vi "desaccade_v2.vi"(10 "Sample Rate":dbl=500.0 format="%.2f", 11 "Velocity Data IN":dbl[][](array[numeric])) -> ()   [LabVIEW 2016]
uses:
  <vilib>/Analysis/3filter.llb/Savitzky-Golay Filter (DBL).vi
  comm.lvlib
  <vilib>/Analysis/NI_AALPro.lvlib
  <vilib>/Analysis/NI_AALBase.lvlib
  <vilib>/Analysis/NI_AAL_SigProc.lvlib
panel:
  out "Waveform Graph 3":dbl[][](graph)
  out "Waveform Graph 2":dbl[](graph)
  out "Waveform Graph":dbl[][](graph)
  in  "Impulse Positions":T1(array[cluster])=[{"Start"=-31, "End"=518, "Impulse Plane"=enum."Other", "Impulse Direction +ve?"=TRUE, "Time offset"=0, "Amplitude offset"=0.0}, {"Start"=369, "End"=913, "Impulse Plane"=enum."Other", "Impulse Direction +ve?"=TRUE, "Time offset"=0, "Amplitude offset"=0.0}, {"Start"=570, "End"=1018, "Impulse Plane"=enum."Other", "Impulse Direction +ve?"=FALSE, "Time offset"=0, "Amplitude offset"=0.0}, {"Start"=770, "End"=1311, "Impulse Plane"=enum."Other", "Impulse Direction +ve?"=TRUE, "Time offset"=0, "Amplitude offset"=0.0}, {"Start"=969, "End"=1417, "Impulse Plane"=enum."Other", "Impulse Direction +ve?"=FALSE, "Time offset"=0, "Amplitude offset"=0.0}, {"Start"=1170, "End"=1708, "Impulse Plane"=enum."Other", "Impulse Direction +ve?"=TRUE, "Time offset"=0, "Amplitude offset"=0.0}, {"Start"=1371, "End"=1819, "Impulse Plane"=enum."Other", "Impulse Direction +ve?"=FALSE, "Time offset"=0, "Amplitude offset"=0.0}, {"Start"=1570, "End"=2104, "Impulse Plane"=enum."Other", "Impulse Direction +ve?"=TRUE, "Time offset"=0, "Amplitude offset"=0.0}, {"Start"=1770, "End"=2218, "Impulse Plane"=enum."Other", "Impulse Direction +ve?"=FALSE, "Time offset"=0, "Amplitude offset"=0.0}, {"Start"=1971, "End"=2508, "Impulse Plane"=enum."Other", "Impulse Direction +ve?"=TRUE, "Time offset"=0, "Amplitude offset"=0.0}, {"Start"=2171, "End"=2619, "Impulse Plane"=enum."Other", "Impulse Direction +ve?"=FALSE, "Time offset"=0, "Amplitude offset"=0.0}, {"Start"=2370, "End"=2917, "Impulse Plane"=enum."Other", "Impulse Direction +ve?"=TRUE, "Time offset"=0, "Amplitude offset"=0.0}, {"Start"=2571, "End"=3019, "Impulse Plane"=enum."Other", "Impulse Direction +ve?"=FALSE, "Time offset"=0, "Amplitude offset"=0.0}, {"Start"=2771, "End"=3308, "Impulse Plane"=enum."Other", "Impulse Direction +ve?"=TRUE, "Time offset"=0, "Amplitude offset"=0.0}, {"Start"=2970, "End"=3418, "Impulse Plane"=enum."Other", "Impulse Direction +ve?"=FALSE, "Time offset"=0, "Amplitude offset"=0.0}, {"Start"=3172, "End"=3715, "Impulse Plane"=enum."Other", "Impulse Direction +ve?"=TRUE, "Time offset"=0, "Amplitude offset"=0.0}, {"Start"=3372, "End"=3820, "Impulse Plane"=enum."Other", "Impulse Direction +ve?"=FALSE, "Time offset"=0, "Amplitude offset"=0.0}, {"Start"=3572, "End"=4107, "Impulse Plane"=enum."Other", "Impulse Direction +ve?"=TRUE, "Time offset"=0, "Amplitude offset"=0.0}, {"Start"=3772, "End"=4220, "Impulse Plane"=enum."Other", "Impulse Direction +ve?"=FALSE, "Time offset"=0, "Amplitude offset"=0.0}, {"Start"=3972, "End"=4512, "Impulse Plane"=enum."Other", "Impulse Direction +ve?"=TRUE, "Time offset"=0, "Amplitude offset"=0.0}, {"Start"=4172, "End"=4620, "Impulse Plane"=enum."Other", "Impulse Direction +ve?"=FALSE, "Time offset"=0, "Amplitude offset"=0.0}, {"Start"=4373, "End"=4920, "Impulse Plane"=enum."Other", "Impulse Direction +ve?"=TRUE, "Time offset"=0, "Amplitude offset"=0.0}, {"Start"=4572, "End"=5020, "Impulse Plane"=enum."Other", "Impulse Direction +ve?"=FALSE, "Time offset"=0, "Amplitude offset"=0.0}, {"Start"=4773, "End"=5315, "Impulse Plane"=enum."Other", "Impulse Direction +ve?"=TRUE, "Time offset"=0, "Amplitude offset"=0.0}, {"Start"=4973, "End"=5421, "Impulse Plane"=enum."Other", "Impulse Direction +ve?"=FALSE, "Time offset"=0, "Amplitude offset"=0.0}, {"Start"=5173, "End"=5716, "Impulse Plane"=enum."Other", "Impulse Direction +ve?"=TRUE, "Time offset"=0, "Amplitude offset"=0.0}, {"Start"=5373, "End"=5821, "Impulse Plane"=enum."Other", "Impulse Direction +ve?"=FALSE, "Time offset"=0, "Amplitude offset"=0.0}, {"Start"=5573, "End"=6110, "Impulse Plane"=enum."Other", "Impulse Direction +ve?"=TRUE, "Time offset"=0, "Amplitude offset"=0.0}, {"Start"=5773, "End"=6221, "Impulse Plane"=enum."Other", "Impulse Direction +ve?"=FALSE, "Time offset"=0, "Amplitude offset"=0.0}, {"Start"=5972, "End"=6515, "Impulse Plane"=enum."Other", "Impulse Direction +ve?"=TRUE, "Time offset"=0, "Amplitude offset"=0.0}, {"Start"=6174, "End"=6622, "Impulse Plane"=enum."Other", "Impulse Direction +ve?"=FALSE, "Time offset"=0, "Amplitude offset"=0.0}, {"Start"=6373, "End"=6913, "Impulse Plane"=enum."Other", "Impulse Direction +ve?"=TRUE, "Time offset"=0, "Amplitude offset"=0.0}, {"Start"=6574, "End"=7022, "Impulse Plane"=enum."Other", "Impulse Direction +ve?"=FALSE, "Time offset"=0, "Amplitude offset"=0.0}, {"Start"=6774, "End"=7314, "Impulse Plane"=enum."Other", "Impulse Direction +ve?"=TRUE, "Time offset"=0, "Amplitude offset"=0.0}, {"Start"=6974, "End"=7422, "Impulse Plane"=enum."Other", "Impulse Direction +ve?"=FALSE, "Time offset"=0, "Amplitude offset"=0.0}, {"Start"=7175, "End"=7712, "Impulse Plane"=enum."Other", "Impulse Direction +ve?"=TRUE, "Time offset"=0, "Amplitude offset"=0.0}, {"Start"=7374, "End"=7822, "Impulse Plane"=enum."Other", "Impulse Direction +ve?"=FALSE, "Time offset"=0, "Amplitude offset"=0.0}, {"Start"=7574, "End"=8111, "Impulse Plane"=enum."Other", "Impulse Direction +ve?"=TRUE, "Time offset"=0, "Amplitude offset"=0.0}, {"Start"=7774, "End"=8222, "Impulse Plane"=enum."Other", "Impulse Direction +ve?"=FALSE, "Time offset"=0, "Amplitude offset"=0.0}, {"Start"=7974, "End"=8518, "Impulse Plane"=enum."Other", "Impulse Direction +ve?"=TRUE, "Time offset"=0, "Amplitude offset"=0.0}, {"Start"=8175, "End"=8623, "Impulse Plane"=enum."Other", "Impulse Direction +ve?"=FALSE, "Time offset"=0, "Amplitude offset"=0.0}, {"Start"=8375, "End"=8920, "Impulse Plane"=enum."Other", "Impulse Direction +ve?"=TRUE, "Time offset"=0, "Amplitude offset"=0.0}, {"Start"=8575, "End"=9023, "Impulse Plane"=enum."Other", "Impulse Direction +ve?"=FALSE, "Time offset"=0, "Amplitude offset"=0.0}, {"Start"=8776, "End"=9315, "Impulse Plane"=enum."Other", "Impulse Direction +ve?"=TRUE, "Time offset"=0, "Amplitude offset"=0.0}, {"Start"=8975, "End"=9423, "Impulse Plane"=enum."Other", "Impulse Direction +ve?"=FALSE, "Time offset"=0, "Amplitude offset"=0.0}, {"Start"=9176, "End"=9715, "Impulse Plane"=enum."Other", "Impulse Direction +ve?"=TRUE, "Time offset"=0, "Amplitude offset"=0.0}, {"Start"=9375, "End"=9823, "Impulse Plane"=enum."Other", "Impulse Direction +ve?"=FALSE, "Time offset"=0, "Amplitude offset"=0.0}, {"Start"=9575, "End"=10110, "Impulse Plane"=enum."Other", "Impulse Direction +ve?"=TRUE, "Time offset"=0, "Amplitude offset"=0.0}]
  in  "Desaccading Parameter":T2={"Threshold 1 [Acc]"=0.0, "Threshold 2 [% of TH1]"=0, "tolerance"=2.0, "Search WD "=0.05757575757575758, " always use TH2"=TRUE, "SD for Outliers"=3.0303030303030303, "Max time [ms]"=50.0, "Min time [ms]"=1.0, "Velocity Threshold"=0.05757575757575758} {"Velocity Threshold" scale=50.0..400.0; "SD for Outliers" scale=0.0..5.0; "Search WD" scale=0.0..0.3; "tolerance" scale=0.0..100.0; "Threshold 2 [% of TH1]" scale=0.0..100.0; "Threshold 1 [Acc]" scale=1.0..40000.0}
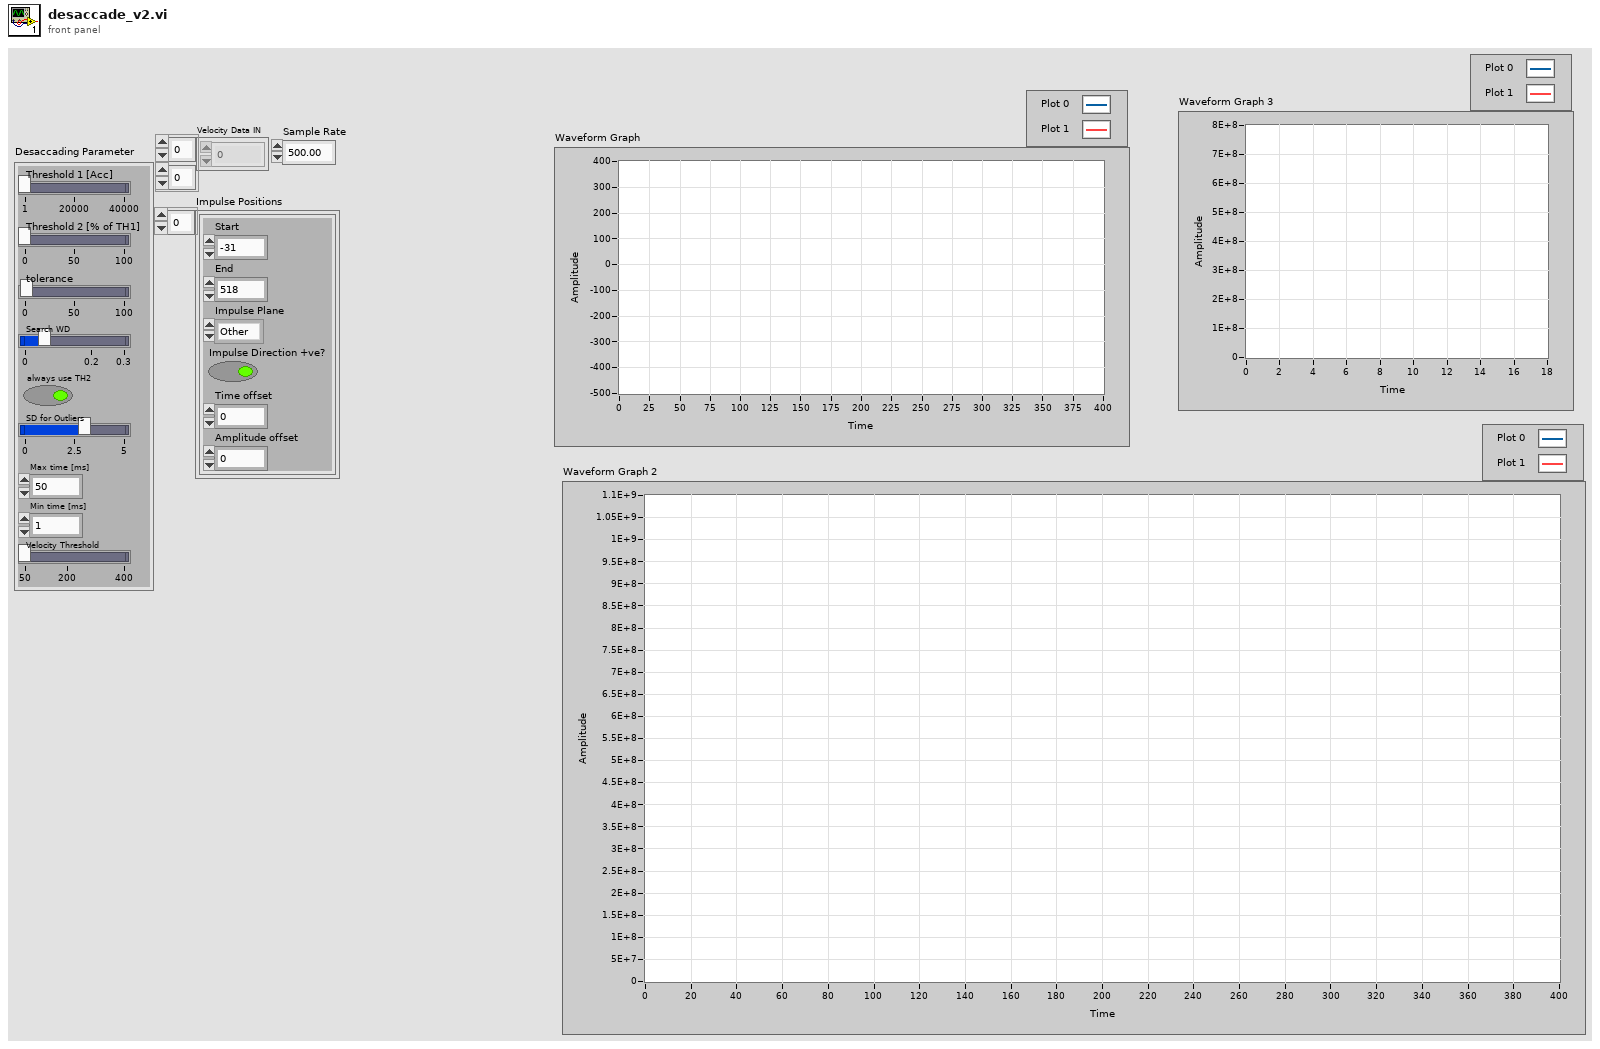
[diagram p1: front panel]
types:
  T1 = cluster{"Start":i32, "End":i32, "Impulse Plane":enum16{"Other", "Yaw", "Pitch", "Roll", "LARP", "RALP"}, "Impulse Direction +ve?":bool, "Time offset":i32, "Amplitude offset":dbl}[]
  T2 = cluster{"Threshold 1 [Acc]":dbl, "Threshold 2 [% of TH1]":i32, "tolerance":dbl, "Search WD ":dbl, " always use TH2":bool, "SD for Outliers":dbl, "Max time [ms]":dbl, "Min time [ms]":dbl, "Velocity Threshold":dbl}
  T3 = cluster{"Raw Acceleration":dbl[], "Smooth Acceleration":dbl[], "Raw Velocity":dbl[], "Smooth Velocity":dbl[]}
  T4 = cluster{"Desaccading Parameter ":cluster{"Threshold 1 [Acc]":dbl, "Threshold 2 [% of TH1]":i32, "tolerance":dbl, "Search WD ":dbl, " always use TH2":bool, "SD for Outliers":dbl, "Max time [ms]":dbl, "Min time [ms]":dbl, "Velocity Threshold":dbl}, "Impulse Positions":cluster{"Start":i32, "End":i32, "Impulse Plane":enum16{"Other", "Yaw", "Pitch", "Roll", "LARP", "RALP"}, "Impulse Direction +ve?":bool, "Time offset":i32, "Amplitude offset":dbl}[], "Velocity Data IN":dbl[][], "Impulse ID":i32, "Sample Rate":dbl, "1D Data":cluster{"Raw Acceleration":dbl[], "Smooth Acceleration":dbl[], "Raw Velocity":dbl[], "Smooth Velocity":dbl[]}, "Datapoint ID":i32, "Saccade Start-End":dbl[]}
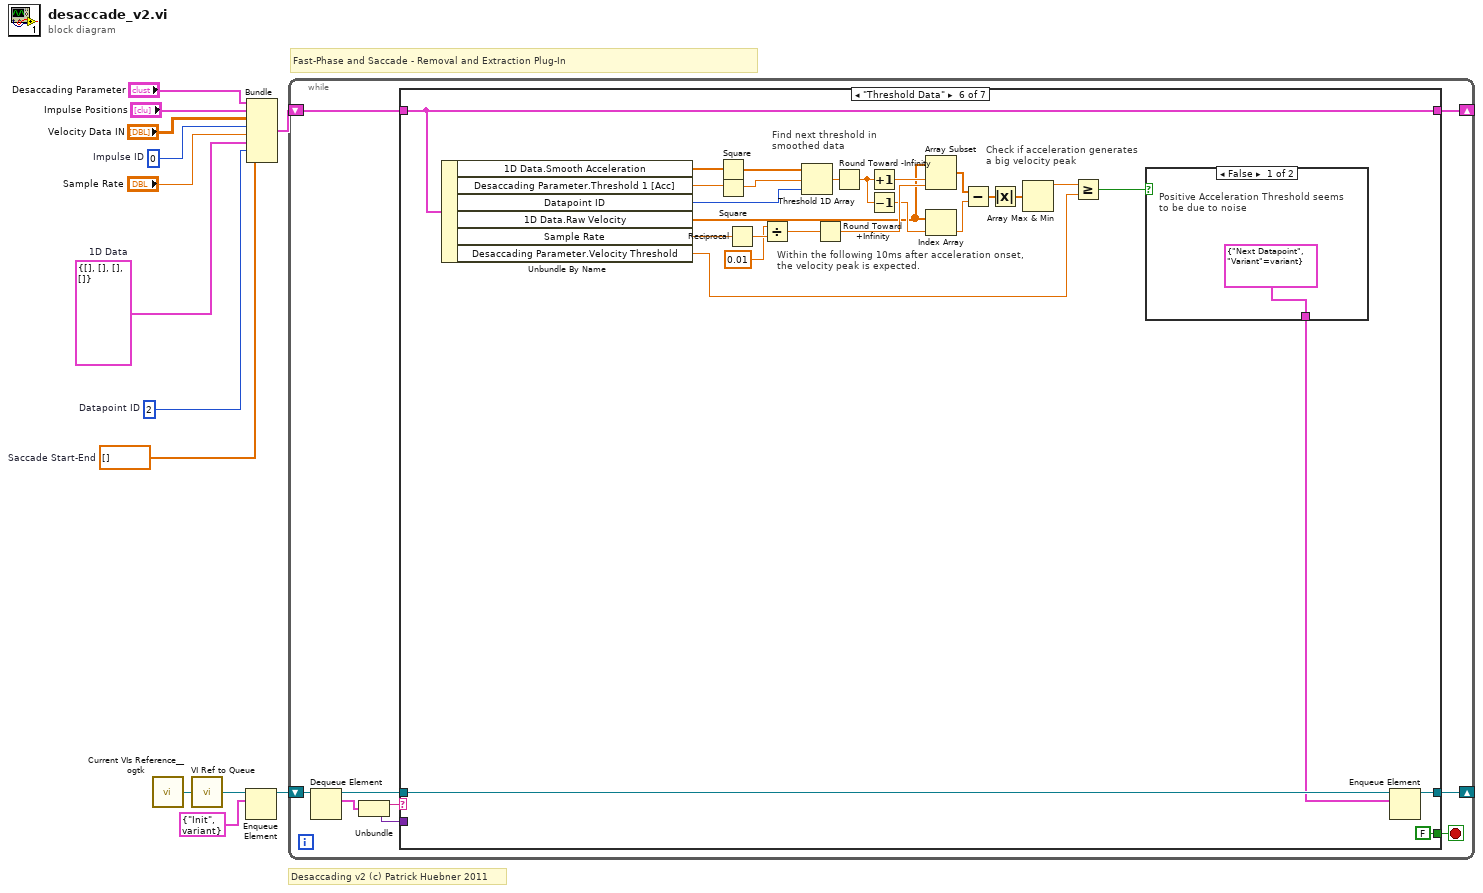
[diagram p0: block diagram]
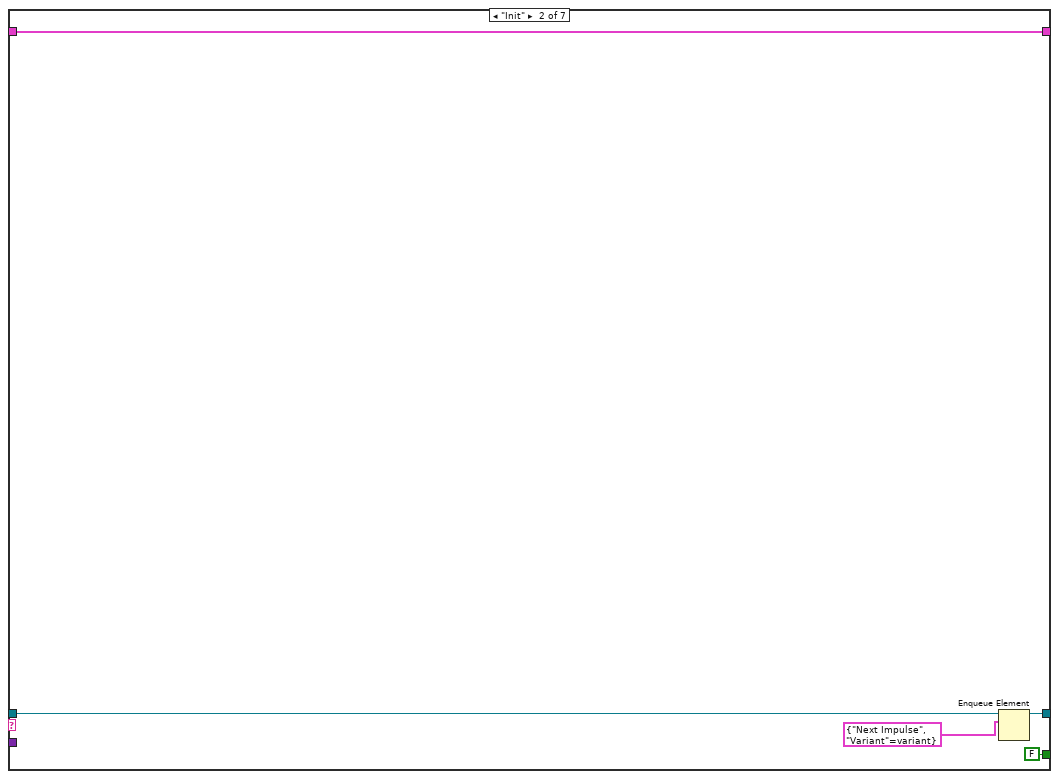
[diagram p3: hidden frame]
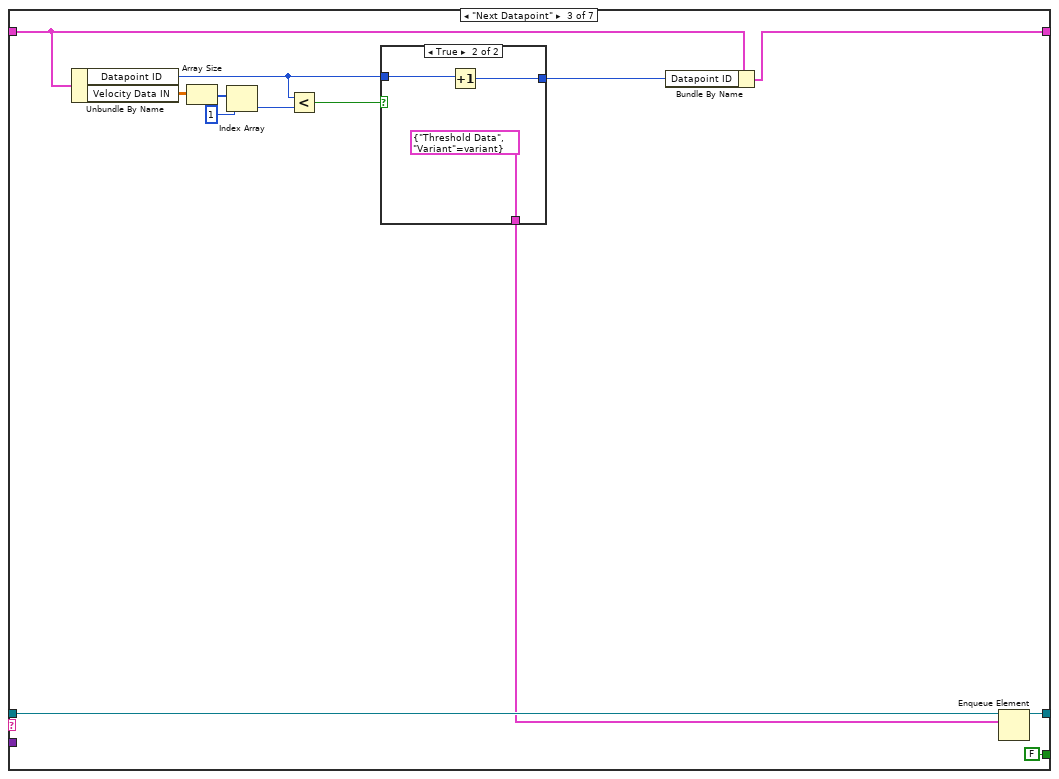
[diagram p4: hidden frame]
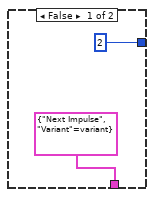
[diagram p5: hidden frame]
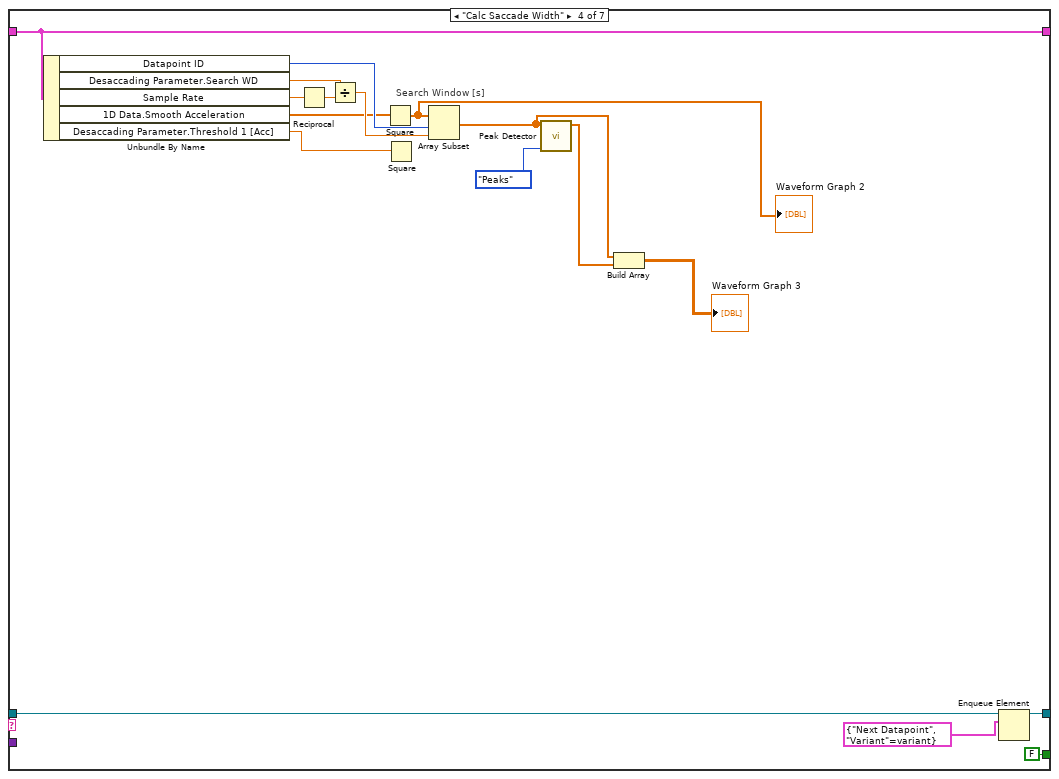
[diagram p6: hidden frame]
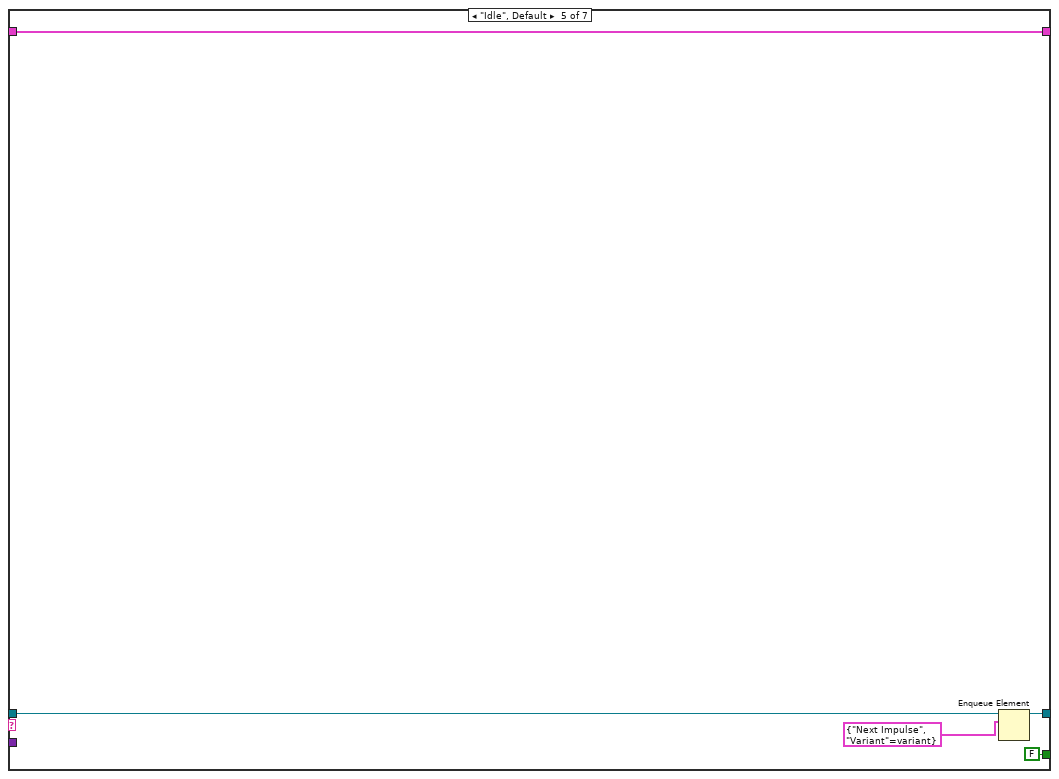
[diagram p7: hidden frame]
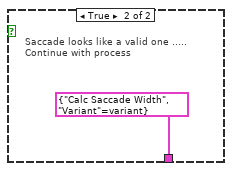
[diagram p8: hidden frame]
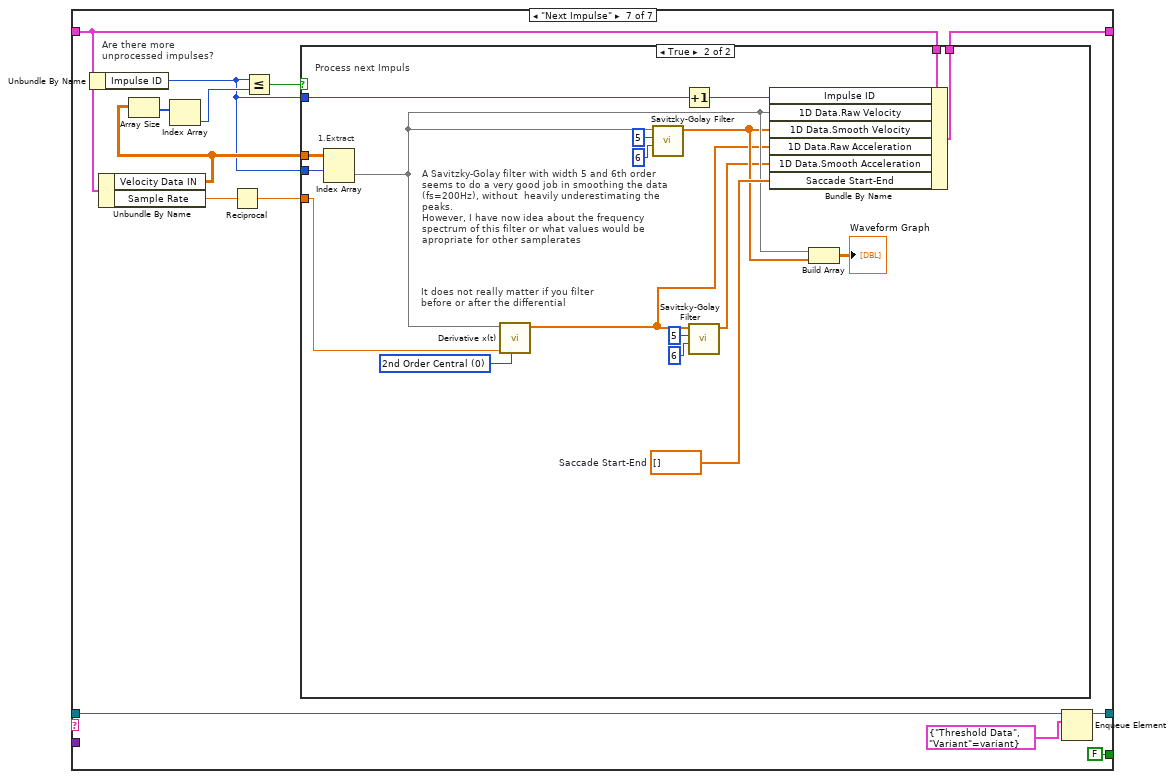
[diagram p9: hidden frame]
diagram:
  w1 = dbl[] []  # Saccade Start-End
  w2 = 2  # Datapoint ID
  w3 = T3 {"Raw Acceleration"=[], "Smooth Acceleration"=[], "Raw Velocity"=[], "Smooth Velocity"=[]}  # 1D Data
  w6 = 0  # Impulse ID
  # "Fast-Phase and Saccade - Removal and Extraction Plug-In"
  # "Desaccading v2 (c) Patrick Huebner 2011"
  n1 = call <userlib>:"Current VIs Reference__ogtk.vi"() -> ("Current VI's reference"=w13:refnum<vi>)  [unwired: 5 in]
  n2 = call "VI Ref to Queue.vi"("VI Refnum"=w13) -> ("queue out"=w12:refnum<queue>)  [unwired: 4 in]
  n3 = Enqueue Element(queue=w12, element=cluster{string, "Variant":variant} {"Init", "Variant"=variant}) -> (queue out=w10:refnum<queue>)  [unwired: 2 in, 2 out]
  n4 = Bundle("Desaccading Parameter"="Desaccading Parameter", "Impulse Positions"="Impulse Positions", "Velocity Data IN"="Velocity Data IN", "Impulse ID"=w6, "Sample Rate"="Sample Rate", "1D Data"=w3, "Datapoint ID"=w2, "Saccade Start-End"=w1) -> (w8:T4)  [unwired: 1 in]
  n5 = while {
    shift-right: [w21] -> _
    shift-left: w10 -> [w22]
    shift-right: [w15] -> _
    shift-left: w8 -> [w14]
    stop <- w16 stop-if-true
    n6 = Dequeue Element(queue=w22) -> (queue out=w20:refnum<queue>, element=w19:cluster{string, "Variant":variant})  [unwired: 2 in, 2 out]
    n7 = Unbundle(w19) -> (w18:string, "Variant"=w17:variant)
    n8 = case shown="\"Threshold Data\"" w18 {
      tunnel: [w24 w29 w42 w64 w69 w96 w111] -> w21
      tunnel: w20 -> [w24 w28 w41 w63 w68 w95 w110]
      tunnel: w17 -> [_ _ _ _ _ _ _]
      tunnel: [_ FALSE FALSE FALSE FALSE FALSE FALSE] -> w16
      tunnel: [w23 w25 w38 w60 w65 w93 w100] -> w15
      tunnel: w14 -> [w23 w25 w39 w60 w65 w93 w101]
      frame "Differentiate" {
      }
      frame "Init" {
        n9 = Enqueue Element(queue=w28, element=cluster{string, "Variant":variant} {"Next Impulse", "Variant"=variant}) -> (queue out=w29:refnum<queue>)  [unwired: 2 in, 2 out]
      }
      frame "Next Datapoint" {
        n10 = Unbundle By Name(w39) -> ("Datapoint ID"=w34:i32, "Velocity Data IN"=w36:dbl[][])
        n11 = Array Size(array=w36) -> (size(s)=w35:i32[])
        n12 = Index Array(array=w35, index=1) -> (element=w33:i32)
        n13 = Less?(x=w34, y=w33) -> (x < y?=w32:bool)
        n14 = case shown="True" w32 {
          tunnel: w34 -> [_ w47]
          tunnel: [2 w46] -> w37
          tunnel: [cluster{string, "Variant":variant} {"Next Impulse", "Variant"=variant} ("element") cluster{string, "Variant":variant} {"Threshold Data", "Variant"=variant} ("element")] -> w31
          frame False {
          }
          frame True {
            n15 = Increment(x=w47) -> (x+1=w46:i32)
          }
        }
        n16 = Bundle By Name(cluster=w39, "Datapoint ID"=w37) -> (w38:T4)
        n17 = Enqueue Element(queue=w41, element=w31) -> (queue out=w42:refnum<queue>)  [unwired: 2 in, 2 out]
      }
      frame "Calc Saccade Width" {
        # "Search Window [s]"
        n18 = Unbundle By Name(w60) -> ("Datapoint ID"=w56:i32, "Desaccading Parameter.Search WD"=w57:dbl, "Sample Rate"=w59:dbl, "1D Data.Smooth Acceleration"=w54:dbl[], "Desaccading Parameter.Threshold 1 [Acc]"=w53:dbl)
        n19 = Reciprocal(x=w59) -> (1/x=w58:dbl)
        n20 = Divide(x=w57, y=w58) -> (x/y=w55:dbl)
        n21 = Square(x=w54) -> (x^2=w51:dbl[])
        "Waveform Graph 2" <- w51
        n22 = Square(x=w53) -> ()  [unwired: 1 out]
        n23 = Array Subset(array=w51, index=w56, length=w55) -> (w49:dbl[])
        n24 = call <vilib>:"Peak Detector.vi"("peaks/valleys"=enum32{"Peaks", "Valleys"}."Peaks", "X"=w49) -> ("Locations"=w48:dbl[])  [unwired: 5 in, 4 out]
        n25 = Build Array(w49, w48) -> (→"Waveform Graph 3":dbl[][])
        n26 = Enqueue Element(queue=w63, element=cluster{string, "Variant":variant} {"Next Datapoint", "Variant"=variant}) -> (queue out=w64:refnum<queue>)  [unwired: 2 in, 2 out]
      }
      frame "Idle", Default {
        n27 = Enqueue Element(queue=w68, element=cluster{string, "Variant":variant} {"Next Impulse", "Variant"=variant}) -> (queue out=w69:refnum<queue>)  [unwired: 2 in, 2 out]
      }
      frame "Threshold Data" {
        # "Check if acceleration generates \na big velocity peak"
        # "Within the following 10ms after acceleration onset, \nthe velocity peak is expected."
        # "Find next threshold in \nsmoothed data"
        n28 = Unbundle By Name(w93) -> ("1D Data.Smooth Acceleration"=w92:dbl[], "Desaccading Parameter.Threshold 1 [Acc]"=w71:dbl, "Datapoint ID"=w89:i32, "1D Data.Raw Velocity"=w80:dbl[], "Sample Rate"=w87:dbl, "Desaccading Parameter.Velocity Threshold"=w74:dbl)
        n29 = Square(x=w92) -> (x^2=w90:dbl[])
        n30 = Square(x=w71) -> (x^2=w70:dbl)
        n31 = Reciprocal(x=w87) -> (1/x=w86:dbl)
        n32 = Divide(x=0.01 ("y"), y=w86) -> (x/y=w84:dbl)
        n33 = Threshold 1D Array(1:w89, 2:w70, 3:w90) -> (0:w91:dbl)
        n34 = Round Toward +Infinity(x=w84) -> (ceil(x): smallest int >= x=w83:dbl)
        n35 = Round Toward -Infinity(1:w91) -> (0:w82:dbl)
        n36 = Increment(x=w82) -> (x+1=w88:dbl)
        n37 = Decrement(x=w82) -> (x-1=w81:dbl)
        n38 = Array Subset(array=w80, index=w88, length=w83) -> (w79:dbl[])
        n39 = Index Array(array=w80, index=w81) -> (element=w78:dbl)
        n40 = Subtract(x=w79, y=w78) -> (x-y=w77:dbl[])
        n41 = Absolute Value(x=w77) -> (abs(x)=w76:dbl[])
        n42 = Array Max & Min(array=w76) -> (max value=w75:dbl)  [unwired: 3 out]
        n43 = Greater Or Equal?(x=w75, y=w74) -> (x >= y?=w73:bool)
        n44 = case shown="False" w73 {
          tunnel: [cluster{string, "Variant":variant} {"Next Datapoint", "Variant"=variant} ("element") cluster{string, "Variant":variant} {"Calc Saccade Width", "Variant"=variant} ("element")] -> w72
          frame False {
            # "Positive Acceleration Threshold seems\nto be due to noise"
          }
          frame True {
            # "Saccade looks like a valid one .....\nContinue with process"
          }
        }
        n45 = Enqueue Element(queue=w95, element=w72) -> (queue out=w96:refnum<queue>)  [unwired: 2 in, 2 out]
      }
      frame "Next Impulse" {
        # "Are there more \nunprocessed impulses?"
        n46 = Unbundle By Name(w101) -> ("Impulse ID"=w99:i32)
        n47 = Unbundle By Name(w101) -> ("Velocity Data IN"=w104:dbl[][], "Sample Rate"=w103:dbl)
        n48 = Array Size(array=w104) -> (size(s)=w107:i32[])
        n49 = Index Array(array=w107) -> (element=w106:i32)  [unwired: 1 in]
        n50 = Reciprocal(x=w103) -> (1/x=w102:dbl)
        n51 = Less Or Equal?(x=w99, y=w106) -> (x <= y?=w105:bool)
        n52 = case shown="True" w105 {
          tunnel: w104 -> [_ w130]
          tunnel: w99 -> [_ w129]
          tunnel: w102 -> [_ w119]
          tunnel: w101 -> [w112 w127]
          tunnel: [w112 w124] -> w100
          tunnel: w99 -> [_ w120]
          frame False {
            # "Done processing"
          }
          frame True {
            w118 = dbl[] []  # Saccade Start-End
            w128 = u16 0 items=["2nd Order Central", "4th Order Central", "Forward", "Backward"] ("method")
            # "A Savitzky-Golay filter with width 5 and 6th order\nseems to do a very good job in smoothing the data\n(fs=200Hz), without  heavily underestimating the \npeaks. \nHowever, I have now idea about the frequency\nspectrum of this filter or what values would be\napropriate for other samplerates"
            # "It does not really matter if you filter \nbefore or after the differential"
            # "1.Extract"
            # "Process next Impuls"
            n53 = Index Array(array=w130, index (row)=w129) -> (element=w116:dbl[])  [unwired: 1 in]
            n54 = call <vilib>:"Derivative x(t).vi"("method"=w128, "dt"=w119, "X"=w116) -> ("dX/dt"=w114:dbl[])  [unwired: 7 in, 1 out]
            n55 = call-poly <vilib>:"Savitzky-Golay Filter.vi"("polynomial order"=6, "side points"=5, "X"=w116) -> ("Filtered X"=w115:dbl[])  [unwired: 7 in, 1 out]
            n56 = Increment(x=w120) -> (x+1=w121:i32)
            n57 = call-poly <vilib>:"Savitzky-Golay Filter.vi"("polynomial order"=6, "side points"=5, "X"=w114) -> ("Filtered X"=w113:dbl[])  [unwired: 7 in, 1 out]
            n58 = Bundle By Name(cluster=w127, "Impulse ID"=w121, "1D Data.Raw Velocity"=w116, "1D Data.Smooth Velocity"=w115, "1D Data.Raw Acceleration"=w114, "1D Data.Smooth Acceleration"=w113, "Saccade Start-End"=w118) -> (w124:T4)
            n59 = Build Array(w116, w115) -> (→"Waveform Graph":dbl[][])
          }
        }
        n60 = Enqueue Element(queue=w110, element=cluster{string, "Variant":variant} {"Threshold Data", "Variant"=variant}) -> (queue out=w111:refnum<queue>)  [unwired: 2 in, 2 out]
      }
    }
  }
